vi "256ptMovingAverage.vi"(10 "Enable?":bool=TRUE, 11 "Raw input":u16) -> (3 "Avg. output":fxp<+,22,12> format="%.9g")   [LabVIEW 2017, in "FPGA functions.lvlib"]
doc: "256-point moving average"
uses:
  FPGA functions.lvlib
  <vilib>/Platform/TimedLoop/XDataNode/wakeup.ctl
  <vilib>/Platform/TimedLoop/XDataNode/XDNodeRunTimeDep.lvlib
  <vilib>/Platform/TimedLoop/XDataNode/nitl_modes.ctl
  <vilib>/Platform/TimedLoop/XDataNode/timing_clust.ctl
  <vilib>/Platform/TimedLoop/XDataNode/XDataNode.xnode
  <vilib>/rvi/FXPMathLib/basic elements/FxpDiscreteDelay/XNode/nifxpmath_DiscreteDelay.xnode
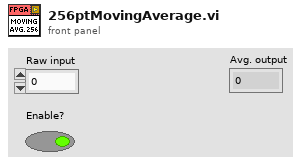
[diagram p1: front panel]
types:
  T1 = typedef "XDNodeRunTimeDep.lvlib/timing_clust.ctl" = cluster{"Expected End [f-1]":u64, "Actual End [f-1]":u64, "Finished Late? [f-1]":bool, "Expected End [i-1]":u64, "Actual End [i-1]":u64, "Finished Late? [i-1]":bool, "Expected Start [i]":u64, "Actual Start [i]":u64, "Expected Start [f]":u64, "Actual Start [f]":u64, "Source Name":string, "Structure Name":string, "Period":i64, "Deadline":i64, "Offset":i64, "Start":i64, "Priority":i32, "Timeout":i32, "Mode":T2, "Wakeup Reason":T3, "Error":errorcluster, "Source Type":string, "Secondary Source Type":string, "Global End Time":u64, "Global Start Time":u64, "Frame Duration":u64, "Iteration Duration":u64, "Assigned CPU":i32, "I/O Scan Engine Mode":u32}
  T2 = typedef "XDNodeRunTimeDep.lvlib/nitl_modes.ctl" = enum32{"No Change", "Process missed periods, maintain original phase", "Discard missed periods, maintain original phase", "Process missed periods, ignore original phase", "Discard missed periods, ignore original phase"}
  T3 = typedef "XDNodeRunTimeDep.lvlib/wakeup.ctl" = enum32{"Normal", "Aborted", "Asynchronous wakeup", "Timing source error", "Timed loop error", "Timeout"}
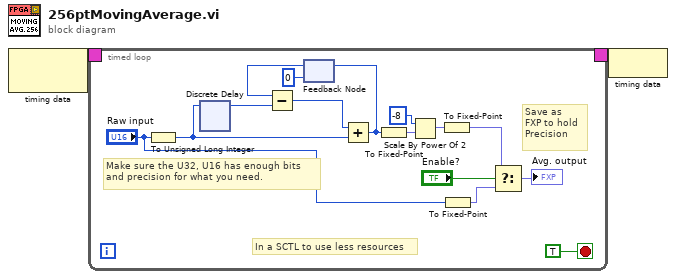
[diagram p0: block diagram]
diagram:
  n1 = node-c288() -> (w2:T1)  [unwired: 1 in]
  n2 = timed-loop {
    timing: w2 -> [_]
    timing-out: [_] -> w1
    stop <- TRUE stop-if-true
    # "Save as \nFXP to hold\nPrecision"
    # "In a SCTL to use less resources"
    # "Make sure the U32, U16 has enough bits \nand precision for what you need."
    n3 = To Unsigned Long Integer(number="Raw input") -> (unsigned 32bit integer=w13:u32)
    n4 = xnode ("Discrete Delay")("D"=w13) -> ("Q"=w16:u32)
    n5 = feedback #1(u32 0) -> (w14:u32)
    n6 = Subtract(x=w14, y=w16) -> (x-y=w15:u32)
    n7 = Add(x=w15, y=w13) -> (x+y=w6:u32)
    n8 = feedback-in #1(w6) -> ()
    n9 = To Fixed-Point(number=w6) -> (fixed-point=w5:fxp<+,32,22>)  [unwired: 1 in]
    n10 = Scale By Power Of 2(n=i16 -8, x=w5) -> (x*2^n=w3:fxp<+,32,22>)
    n11 = To Fixed-Point(number=w3) -> (fixed-point=w4:fxp<+,22,12>)  [unwired: 1 in]
    n12 = To Fixed-Point(number="Raw input") -> (fixed-point=w9:fxp<+,22,12>)  [unwired: 1 in]
    n13 = Select(t=w4, s="Enable?", f=w9) -> (s? t:f=→"Avg. output":fxp<+,22,12>)
  }
  n14 = node-c288(w1) -> ()
